vi "Keithley 2220A 2230A 2231A Measure Voltage.vi"(8 "error in (no error)":errorcluster, 11 "VISA resource name":refnum<visa-resource-name>) -> (0 "error out":errorcluster, 2 "Measured Voltage":sgl, 3 "VISA resource name out":refnum<visa-resource-name>)   [LabVIEW 2019]
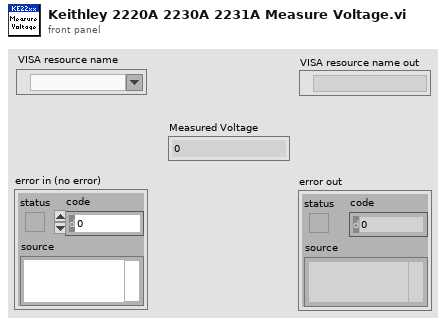
[diagram p1: front panel]
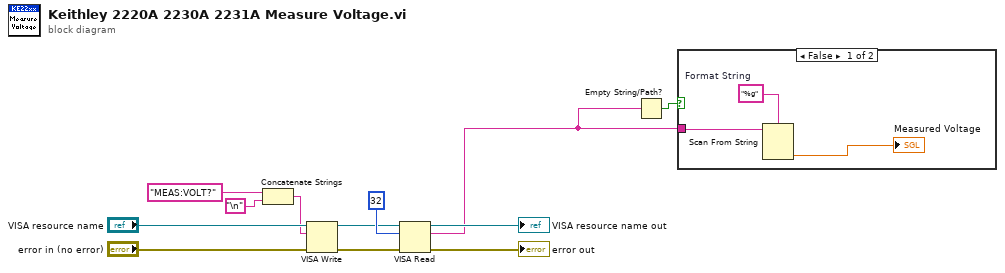
[diagram p0: block diagram]
diagram:
  n1 = Concatenate Strings("MEAS:VOLT?" ("format string"), "\n") -> (w9:string)
  n2 = VISA Write(VISA resource name="VISA resource name", write buffer=w9, error in (no error)="error in (no error)") -> (VISA resource name out=w6:refnum<visa-resource-name>, error out=w5:errorcluster)  [unwired: 1 out]
  n3 = VISA Read(VISA resource name=w6, byte count=u32 32, error in (no error)=w5) -> (VISA resource name out=→"VISA resource name out":refnum<visa-resource-name>, read buffer=w1:string, error out=→"error out":errorcluster)  [unwired: 1 out]
  n4 = Empty String/Path?(string/path=w1) -> (empty?=w2:bool)
  n5 = case shown="False" w2 {
    tunnel: w1 -> [w14 _]
    frame False {
      w15 = "%g"  # Format String
      n6 = Scan From String(format string=w15, input string=w14) -> (output 1=→"Measured Voltage":sgl)  [unwired: 3 in, 3 out]
    }
    frame True {
    }
  }
